vi "Get Server Stop UE.vi"(11 "OOP Server in":refnum<class "OCV2.lvclass">) -> (2 "Server Stop UE":refnum<user-event>, 3 "OOP Server out":refnum<class "OCV2.lvclass">)   [LabVIEW 2019, in "OCV2.lvlib" / "OCV2.lvclass"]
uses:
  OCV2.lvclass
  OCV2.lvclass/OCV2.ctl
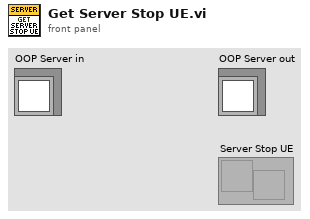
[diagram p1: front panel]
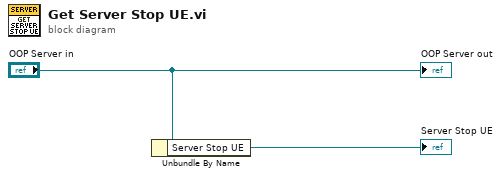
[diagram p0: block diagram]
diagram:
  n1 = Unbundle By Name("OOP Server in") -> ("Server Stop UE"=→"Server Stop UE":refnum<user-event>)
  "OOP Server out" <- "OOP Server in"
